vi "TestLecture.vi"() -> ()   [LabVIEW 2022 SP3]
panel:
  out "array w/ subset deleted":dbl[][](array[numeric])
  out "text":string
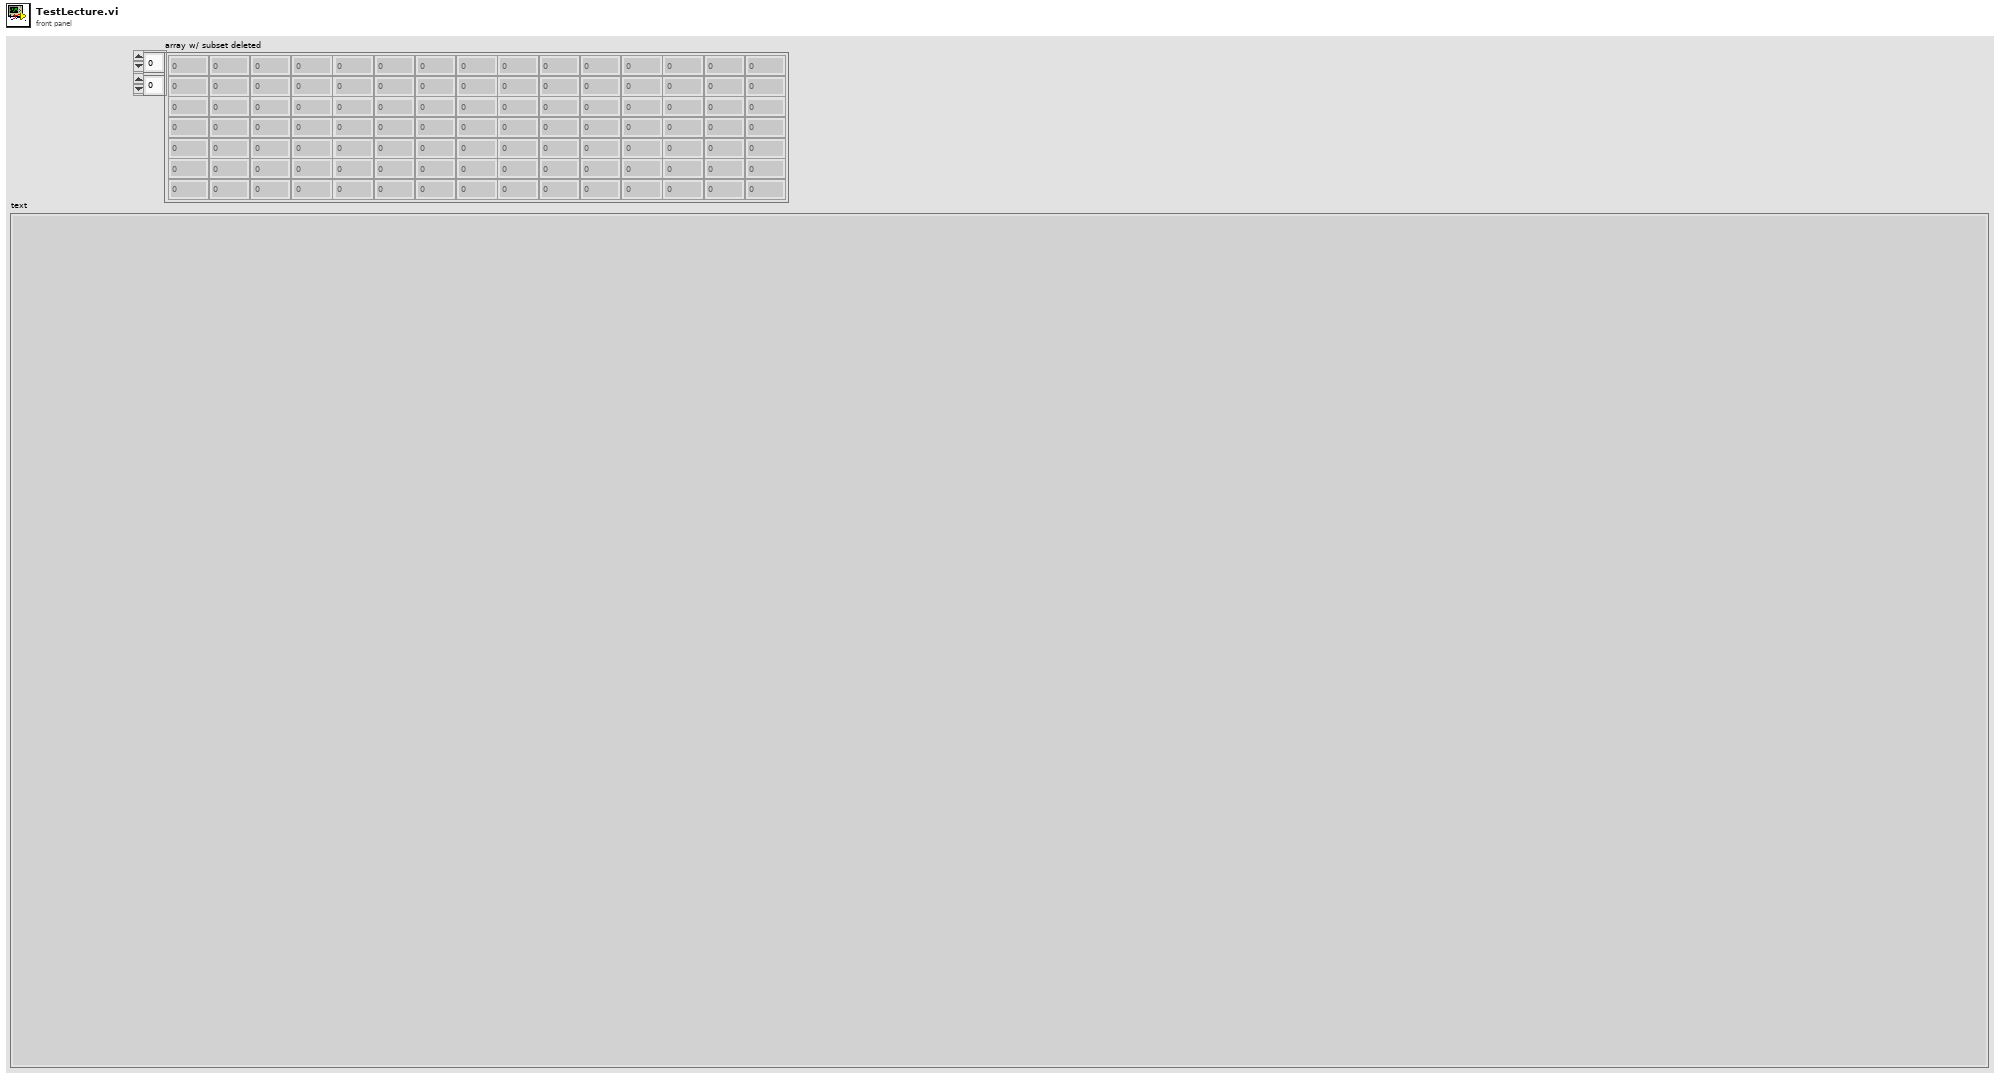
[diagram p1: front panel]
types:
  T1 = enum16{"open", "replace", "create", "open or create", "replace or create", "replace or create with confirmation"}
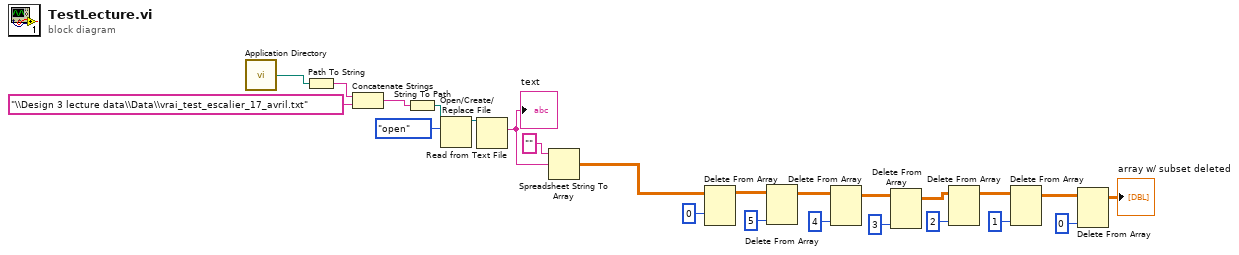
[diagram p0: block diagram]
diagram:
  n1 = call <vilib>:"Application Directory.vi"() -> ("Application Directory"=w24:path)
  n2 = Path To String(path=w24) -> (string=w23:string)
  n3 = Concatenate Strings(w23, "\\Design 3 lecture data\\Data\\vrai_test_escalier_17_avril.txt" ("string")) -> (w21:string)
  n4 = String To Path(string=w21) -> (path=w20:path)
  n5 = Open/Create/Replace File(file path (use dialog)=w20, operation (0:open)=T1."open") -> (refnum out=w18:refnum<file>)  [unwired: 4 in, 2 out]
  n6 = Read from Text File(file (use dialog)=w18) -> (text=w17:string)  [unwired: 3 in, 3 out]
  "text" <- w17
  n7 = Spreadsheet String To Array(format string="", spreadsheet string=w17) -> (array=w1:dbl[][])  [unwired: 2 in]
  n8 = Delete From Array(array=w1, index (row)=0) -> (array with subset deleted=w14:dbl[][])  [unwired: 2 in, 1 out]
  n9 = Delete From Array(array=w14, index (col)=5 ("disabled index (col)")) -> (array with subset deleted=w12:dbl[][])  [unwired: 2 in, 1 out]
  n10 = Delete From Array(array=w12, index (col)=4 ("disabled index (col)")) -> (array with subset deleted=w10:dbl[][])  [unwired: 2 in, 1 out]
  n11 = Delete From Array(array=w10, index (col)=3 ("disabled index (col)")) -> (array with subset deleted=w7:dbl[][])  [unwired: 2 in, 1 out]
  n12 = Delete From Array(array=w7, index (col)=2) -> (array with subset deleted=w6:dbl[][])  [unwired: 2 in, 1 out]
  n13 = Delete From Array(array=w6, index (col)=1 ("disabled index (col)")) -> (array with subset deleted=w3:dbl[][])  [unwired: 2 in, 1 out]
  n14 = Delete From Array(array=w3, index (col)=0) -> (array with subset deleted=→"array w/ subset deleted":dbl[][])  [unwired: 2 in, 1 out]
